vi "Select_Network.vi"(11 "base path":path) -> (0 "error out":errorcluster, 1 "SimPars":T1, 2 "CNN Left":refnum<class "CNN.lvclass">, 3 "CNN Right":refnum<class "CNN.lvclass">)   [LabVIEW 2016]
uses:
  biCNN/CNN.lvclass
  biCNN/CNN.lvclass/CNN.ctl
  <vilib>/Utility/xml.llb/Read From XML File.vi
  <vilib>/Utility/xml.llb/Read From XML File(string).vi
  biCNN/AER/AER.lvclass
panel:
  in  "run":bool
  in  "Existing Grids in Results/ 2":i32(listbox)
  out "preview 2":string
  out "preview":string
  in  "Existing Grids in Results/":i32(listbox)
  in  "AERs for LEFT":i32(listbox)
  in  "AERs for RIGHT":i32(listbox)
  # "Select the Networks"
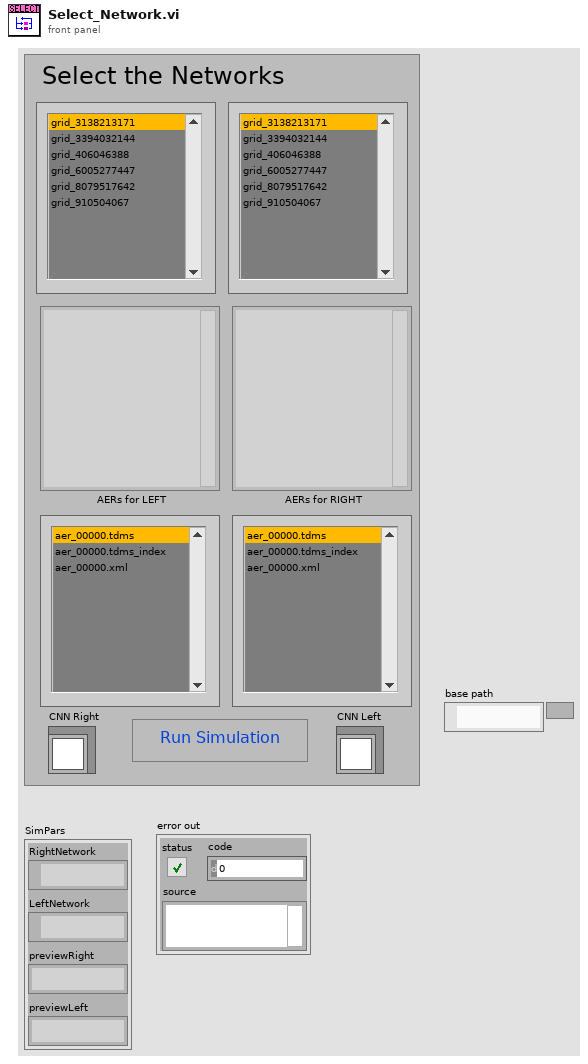
[diagram p1: front panel]
types:
  T1 = cluster{"RightNetwork":path, "LeftNetwork":path, "previewRight":string, "previewLeft":string}
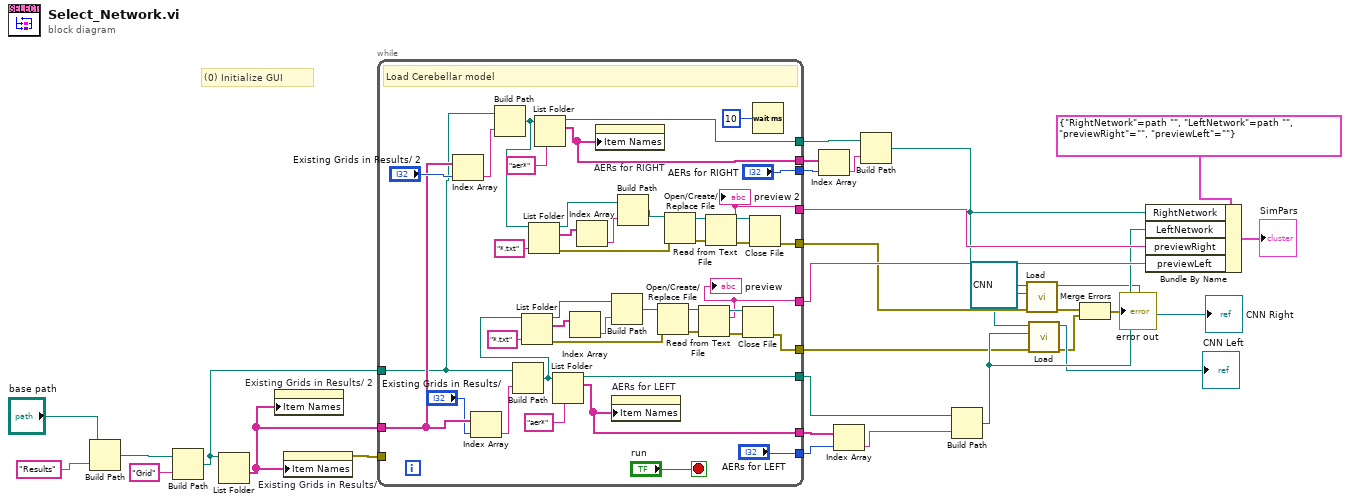
[diagram p0: block diagram]
diagram:
  w8 = refnum<class "CNN.lvclass"> refnum ("CNN in")
  # "(0) Initialize GUI"
  n1 = Build Path(base path="base path", name or relative path="Results") -> (appended path=w27:path)
  n2 = Build Path(base path=w27, name or relative path="Grid") -> (appended path=w25:path)
  n3 = List Folder(path=w25) -> (folder names=w24:string[])  [unwired: 3 in, 3 out]
  n4 = property on="Existing Grids in Results/ 2" class="LstBox (strict)"("Item Names"=w24) -> ()  [unwired: 2 in, 2 out]
  n5 = property on="Existing Grids in Results/" class="LstBox (strict)"("Item Names"=w24) -> (error out=w26:errorcluster)  [unwired: 2 in, 1 out]
  n6 = while {
    tunnel: w26 -> [_]
    tunnel: w24 -> [w66]
    tunnel: w25 -> [w64]
    tunnel: [w69] -> w18
    tunnel: [w39] -> w19
    tunnel: [w38] -> w23
    tunnel: [w37] -> w21
    tunnel: ["AERs for LEFT"] -> w17
    tunnel: ["AERs for RIGHT"] -> w16
    tunnel: [w33] -> w12
    tunnel: [w32] -> w13
    tunnel: [w31] -> w9
    tunnel: [w30] -> w6
    stop <- "run" stop-if-true
    # "Load Cerebellar model"
    n7 = Index Array(array=w66, index="Existing Grids in Results/ 2") -> (element=w65:string)
    n8 = Index Array(array=w66, index="Existing Grids in Results/") -> (element=w71:string)
    n9 = Build Path(base path=w64, name or relative path=w65) -> (appended path=w56:path)
    n10 = Build Path(base path=w64, name or relative path=w71) -> (appended path=w45:path)
    n11 = List Folder(path=w45, pattern="*.txt") -> (path out=w42:path, filenames=w50:string[], error out=w48:errorcluster)  [unwired: 2 in, 1 out]
    n12 = List Folder(path=w56, pattern="*.txt") -> (path out=w53:path, filenames=w54:string[], error out=w57:errorcluster)  [unwired: 2 in, 1 out]
    n13 = List Folder(path=w56, pattern="aer*") -> (path out=w37:path, filenames=w38:string[])  [unwired: 2 in, 2 out]
    n14 = List Folder(path=w45, pattern="aer*") -> (path out=w69:path, filenames=w39:string[])  [unwired: 2 in, 2 out]
    n15 = Index Array(array=w50) -> (element=w43:string)  [unwired: 1 in]
    n16 = Index Array(array=w54) -> (element=w52:string)  [unwired: 1 in]
    n17 = property on="AERs for RIGHT" class="LstBox (strict)"("Item Names"=w38) -> ()  [unwired: 2 in, 2 out]
    n18 = Build Path(base path=w42, name or relative path=w43) -> (appended path=w44:path)
    n19 = property on="AERs for LEFT" class="LstBox (strict)"("Item Names"=w39) -> ()  [unwired: 2 in, 2 out]
    n20 = Build Path(base path=w53, name or relative path=w52) -> (appended path=w51:path)
    n21 = Open/Create/Replace File(file path (use dialog)=w44, error in=w48) -> (refnum out=w40:refnum<file>, error out=w46:errorcluster)  [unwired: 4 in, 1 out]
    n22 = Open/Create/Replace File(file path (use dialog)=w51, error in=w57) -> (refnum out=w62:refnum<file>, error out=w63:errorcluster)  [unwired: 4 in, 1 out]
    n23 = Read from Text File(file (use dialog)=w40, error in=w46) -> (refnum out=w41:refnum<file>, text=w33:string, error out=w47:errorcluster)  [unwired: 2 in, 1 out]
    "preview" <- w33
    n24 = Read from Text File(file (use dialog)=w62, error in=w63) -> (refnum out=w60:refnum<file>, text=w32:string, error out=w61:errorcluster)  [unwired: 2 in, 1 out]
    "preview 2" <- w32
    n25 = Close File(refnum=w41, error in=w47) -> (error out=w30:errorcluster)  [unwired: 1 out]
    n26 = Close File(refnum=w60, error in=w61) -> (error out=w31:errorcluster)  [unwired: 1 out]
    n27 = Wait (ms)(milliseconds to wait=u32 10) -> ()  [unwired: 1 out]
  }
  n28 = Index Array(array=w23, index=w16) -> (element=w22:string)
  n29 = Index Array(array=w19, index=w17) -> (element=w20:string)
  n30 = Build Path(base path=w21, name or relative path=w22) -> (appended path=w10:path)
  n31 = Build Path(base path=w18, name or relative path=w20) -> (appended path=w7:path)
  n32 = call "Load.vi"("error in (no error)"=w9, "AER path"=w10, "CNN in"=w8) -> ("error out"=w3:errorcluster, "CNN out"=→"CNN Right":refnum<class "CNN.lvclass">)  [unwired: 7 in]
  n33 = call "Load.vi"("error in (no error)"=w6, "AER path"=w7, "CNN in"=w8) -> ("error out"=w2:errorcluster, "CNN out"=→"CNN Left":refnum<class "CNN.lvclass">)  [unwired: 7 in]
  n34 = Merge Errors(w3, w2) -> (→"error out":errorcluster)
  n35 = Bundle By Name(cluster=T1 {"RightNetwork"=path "", "LeftNetwork"=path "", "previewRight"="", "previewLeft"=""}, "RightNetwork"=w10, "LeftNetwork"=w7, "previewRight"=w13, "previewLeft"=w12) -> (→"SimPars":T1)
